vi "8.9.-Momento h6.vi"(1 "n20/n02/n11/n30/n12/n21/n03":dbl[](array[numeric])) -> (0 "M6":dbl)   [LabVIEW 2020]
panel:
  # "Visión Artificial - Momentos Invariantes de Hu\nDiego Cervantes Rodríguez\ndicer0.com"
  # "M6 = ((n20-n02)*((n30+n12)^2 -(n21+n03)^2)))+((4*n11)*(n30+n12)*(n21+n03))"
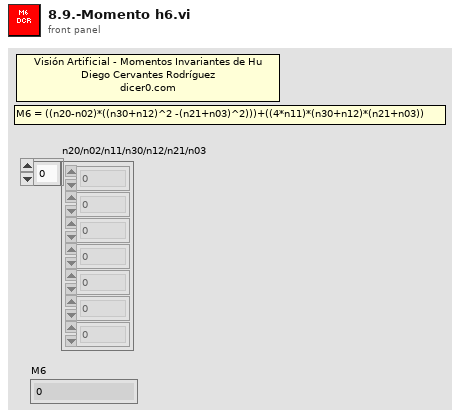
[diagram p1: front panel]
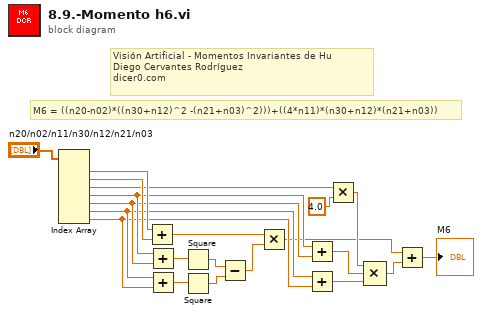
[diagram p0: block diagram]
diagram:
  # "Visión Artificial - Momentos Invariantes de Hu\nDiego Cervantes Rodríguez\ndicer0.com"
  # "M6 = ((n20-n02)*((n30+n12)^2 -(n21+n03)^2)))+((4*n11)*(n30+n12)*(n21+n03))"
  n1 = Index Array(array="n20/n02/n11/n30/n12/n21/n03") -> (element #1=w20:dbl, element #2=w19:dbl, element #3=w11:dbl, element #4=w10:dbl, element #5=w9:dbl, element #6=w8:dbl, element #7=w7:dbl)  [unwired: 7 in]
  n2 = Add(x=w20, y=w19) -> (x+y=w13:dbl)
  n3 = Add(x=w10, y=w9) -> (x+y=w18:dbl)
  n4 = Add(x=w8, y=w7) -> (x+y=w17:dbl)
  n5 = Square(x=w18) -> (x^2=w16:dbl)
  n6 = Square(x=w17) -> (x^2=w15:dbl)
  n7 = Subtract(x=w16, y=w15) -> (x-y=w14:dbl)
  n8 = Multiply(x=w13, y=w14) -> (x*y=w3:dbl)
  n9 = Add(x=w10, y=w9) -> (x+y=w6:dbl)
  n10 = Add(x=w8, y=w7) -> (x+y=w4:dbl)
  n11 = Multiply(x=w11, y=4.0) -> (x*y=w5:dbl)
  n12 = Compound Arithmetic op=MULTIPLY(w5, w6, w4) -> (w2:dbl)
  n13 = Add(x=w3, y=w2) -> (x+y=→"M6":dbl)
